vi "solar_voy TCP Open.vi"(6 "IP Address":string, 7 "Instance":i32, 8 "error in (no error)":errorcluster, 9 "timeout ms (-1)":i32=-1, 10 "Port":u16, 11 "Voyager Refnum in":T1) -> (0 "error out":errorcluster, 2 "Connection ID":refnum<k5>, 3 "Voyager Refnum out":T1)   [LabVIEW 2018]
doc: "This opens a TCP connection to a server. The client port is randomly assigned."
uses:
  solar_voy_ctl Voyager Refnum.ctl
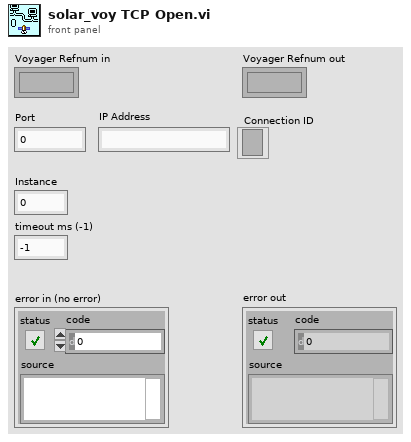
[diagram p1: front panel]
types:
  T1 = typedef "solar_voy_ctl Voyager Refnum.ctl" = refnum<k1>
  T2 = typedef "solar_voy_ctl Voyager.ctl" = cluster{"PACKETS":T3[], "COSMOS_Root":path, "CMD_HDR":T8, "TLM_HDR":T8, "TCPs":T9[], "VoyagerIDOffset":cluster{"VoyagerIDOffset":u16[], "Target Names":string[]}}
  T3 = typedef "solar_voy_def_ctl PACKET.ctl" = cluster{"PACKET_ID":T4, "ENDIAN":enum8{"BIG", "LITTLE"}, "DESC":string, "HZRD":bool, "ITEMS":T5[], "NoExport":bool, "last_time":timestamp, "last_count":u32, "last_data":string}
  T4 = typedef "solar_voy_def_ctl PACKET_ID.ctl" = cluster{"ID":u16, "CMD":enum8{"CMD", "TLM"}, "TARGET":string, "PACKET":string}
  T5 = typedef "solar_voy_def_ctl ITEM.ctl" = cluster{"NAME":string, "OFFSET":i32, "SIZE":i32, "TYPE":T6, "EACH_SIZE":i32, "LVTYPE":T7, "MIN":dbl, "MAX":dbl, "DEFAULT":string, "DESC":string, "ID":bool, "MODIFIERS":variant, "last_value":variant}
  T6 = typedef "solar_voy_def_ctl ITEM TYPE.ctl" = enum8{"BLOCK", "INT", "UINT", "FLOAT", "STRING"}
  T7 = typedef "solar_type Item Type.ctl" = enum16{"NULL", "UNKNOWN", "CLUSTER", "I8", "I16", "I32", "I64", "U8", "U16", "U32", "U64", "U8_ENUM", "U16_ENUM", "U32_ENUM", "SGL", "DBL", "BOOLEAN", "STRING", "PATH", "VISA", "TAG", "TIME", "I8_1D", "I16_1D", "I32_1D", "I64_1D", "U8_1D", "U16_1D", "U32_1D", "U64_1D", "U8_ENUM_1D", "U16_ENUM_1D", "U32_ENUM_1D", "SGL_1D", "DBL_1D", "BOOLEAN_1D", "STRING_1D", "PATH_1D", "VISA_1D", "TAG_1D", "TIME_1D", "I8_2D", "I16_2D", "I32_2D", "I64_2D", "U8_2D", "U16_2D", "U32_2D", "U64_2D", "U8_ENUM_2D", "U16_ENUM_2D", "U32_ENUM_2D", "SGL_2D", "DBL_2D", "BOOLEAN_2D", "STRING_2D", "PATH_2D", "VISA_2D", "TAG_2D", "TIME_2D"}
  T8 = typedef "solar_voy_def_ctl HDR.ctl" = cluster{"ITEMS":T5[], "LENGTH_NAME":string, "LENGTH_VALUE_OFFSET":i32, "ID_NAME":string, "ENDIAN":enum8{"BIG", "LITTLE"}, "GUID_NAME":string, "DEFAULT_TARGET":string, "DEFAULT_PACKET":string, "DEFAULT_ERROR":string}
  T9 = typedef "solar_voy_ctl TCP.ctl" = cluster{"Connected":bool, "Port":u16, "Listener":refnum<k5>, "ServerIP":string, "TCP":refnum<k5>, "Setup":T10, "VIRefnum":refnum<vi>, "TARGETS_CMD":string[], "TARGETS_TLM":string[]}
  T10 = typedef "solar_voy_ctl Port Setup.ctl" = enum8{"SERVER", "CLIENT", "SERVER_CMD", "SERVER_TLM"}
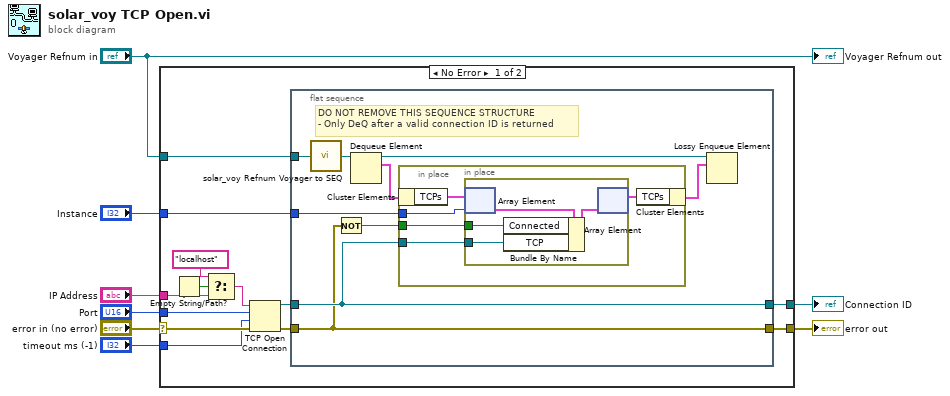
[diagram p0: block diagram]
diagram:
  n1 = case shown="No Error" "error in (no error)" {
    selector: "error in (no error)" -> [w17 w40]
    tunnel: [w21 _] -> w8
    tunnel: "Instance" -> [w20 _]
    tunnel: [w19 w40] -> w5
    tunnel: "Voyager Refnum in" -> [w18 _]
    tunnel: "timeout ms (-1)" -> [w14 _]
    tunnel: "IP Address" -> [w11 _]
    tunnel: "Port" -> [w13 _]
    frame No Error {
      n2 = Empty String/Path?(string/path=w11) -> (empty?=w12:bool)
      n3 = Select(t="localhost", s=w12, f=w11) -> (s? t:f=w10:string)
      n4 = TCP Open Connection(address=w10, remote port or service name=w13, timeout ms (60000)=w14, error in (no error)=w17) -> (connection ID=w15:refnum<k5>, error out=w16:errorcluster)  [unwired: 1 in]
      n5 = flat-sequence {
        tunnel: w15 -> [w26]
        tunnel: w20 -> [w30]
        tunnel: w18 -> [w27]
        tunnel: w16 -> [w25]
        tunnel: [w25] -> w19
        tunnel: [w26] -> w21
        frame #0 {
          # "DO NOT REMOVE THIS SEQUENCE STRUCTURE\n- Only DeQ after a valid connection ID is returned"
          n6 = call "solar_voy Refnum Voyager to SEQ.vi"("Voyager Refnum"=w27) -> ("Voyager SEQ"=w29:refnum<queue>)
          n7 = Not(x=w25) -> (.not. x?=w24:bool)
          n8 = Dequeue Element(queue=w29) -> (queue out=w28:refnum<queue>, element=w23:T2)  [unwired: 2 in, 2 out]
          n9 = in-place {
            in-place-border: w30 -> [w35]
            in-place-border: w26 -> [w34]
            in-place-border: w24 -> [w33]
            n10 = in-place-cluster #1(w23) -> ("TCPs"=w32:T9[])
            n11 = in-place {
              in-place-border: w34 -> [w37]
              in-place-border: w33 -> [w36]
              n12 = in-place-array #2(w32, w35) -> (w39:T9)
              n13 = Bundle By Name(cluster=w39, "Connected"=w36, "TCP"=w37) -> (w38:T9)
              n14 = in-place-array #2(w38) -> (w31:T9[])  [unwired: 1 out]
            }
            n15 = in-place-cluster #1("TCPs"=w31) -> (w22:T2)
          }
          n16 = Lossy Enqueue Element(queue=w28, element=w22) -> ()  [unwired: 1 in, 4 out]
        }
      }
    }
    frame Error {
    }
  }
  "Connection ID" <- w8
  "error out" <- w5
  "Voyager Refnum out" <- "Voyager Refnum in"
